vi "Stop Core.vi"(10 "final error code":i32, 11 "TestSetup in":refnum<class "TestSetup.lvclass">) -> (3 "TestSetup out":refnum<class "TestSetup.lvclass">)   [LabVIEW 2019, in "TestSetup.lvlib" / "TestSetup.lvclass"]
uses:
  TestSetup.lvclass
  TestSetup.lvclass/TestSetup.ctl
  SystemSetup/SystemSetup/SystemSetup.lvclass
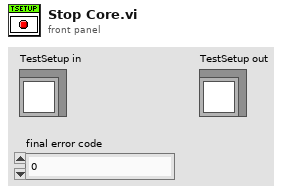
[diagram p1: front panel]
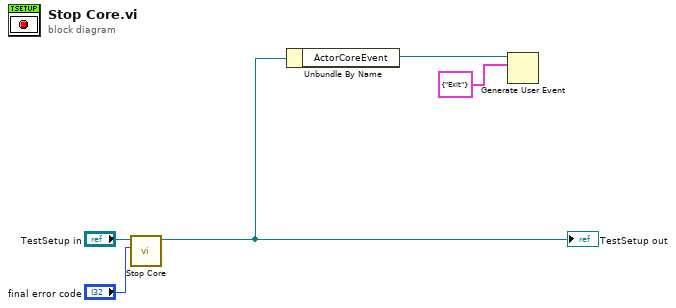
[diagram p0: block diagram]
diagram:
  n1 = call-parent "Stop Core.vi"("final error code"="final error code", "Event Source In"="TestSetup in") -> ("Event Source Out"=w3:refnum<class "TestSetup.lvclass">)  [unwired: 9 in]
  "TestSetup out" <- w3
  n2 = Unbundle By Name(w3) -> ("ActorCoreEvent"=w2:refnum<user-event>)
  n3 = Generate User Event(user event=w2, event data cluster=cluster{"ActorCoreMessage":string} {"ActorCoreMessage"="Exit"} ("event data")) -> ()  [unwired: 2 in, 2 out]
